vi "Utility_Read_Fluid_XML.vi"(11 "path":string) -> (3 "xmlout":string)   [LabVIEW 2016]
doc: "Reads pure fluid names from files in a given directory."
panel:
  out "Pure Fluids in REFPROP":string[][](table)=[["butene", "1-butene"], ["acetone", "propanone"], ["ammonia", "ammonia"], ["argon", "argon"], ["benzene", "benzene"], ["butane", "n-butane"], ["dodecane", "dodecane"], ["cis-butene", "cis-2-butene"], ["perfluorobutane", "decafluorobutane"], ["perfluoropentane", "dodecafluoropentane"], ["trifluoroiodomethane", "trifluoroiodomethane"], ["carbon monoxide", "carbon monoxide"], ["carbon dioxide", "carbon dioxide"], ["carbonyl sulfide", "carbon oxide sulfide"], ["cyclohexane", "cyclohexane"], ["cyclopropane", "cyclopropane"], ["deuterium", "deuterium"], ["heavy water", "deuterium oxide"], ["decane", "decane"], ["dimethylether", "ethylene oxide"], ["ethane", "ethane"], ["ethanol", "ethyl alcohol"], ["ethylene", "ethene"], ["fluorine", "fluorine"], ["hydrogen sulfide", "hydrogen sulfide"], ["helium", "helium-4"], ["heptane", "heptane"], ["hexane", "hexane"], ["hydrogen (normal)", "hydrogen (normal)"], ["isobutene", "2-methyl-1-propene"], ["isohexane", "2-methylpentane"], ["isopentane", "2-methylbutane"], ["isobutane", "2-methylpropane"], ["krypton", "krypton"], ["methane", "methane"], ["methanol", "methanol"], ["nitrous oxide", "dinitrogen monoxide"], ["neon", "neon"], ["neopentane", "2,2-dimethylpropane"], ["nitrogen trifluoride", "nitrogen trifluoride"], ["nitrogen", "nitrogen"], ["nonane", "nonane"], ["octane", "octane"], ["oxygen", "oxygen"], ["parahydrogen", "parahydrogen"], ["pentane", "pentane"], ["propane", "propane"], ["propylene", "propene"], ["propyne", "propyne"], ["R11", "trichlorofluoromethane"], ["R113", "1,1,2-trichloro-1,2,2-trifluoroethane"], ["R114", "1,2-dichloro-1,1,2,2-tetrafluoroethane"], ["R115", "chloropentafluoroethane"], ["R116", "hexafluoroethane"], ["R12", "dichlorodifluoromethane"], ["R123", "2,2-dichloro-1,1,1-trifluoroethane"], ["R124", "1-chloro-1,2,2,2-tetrafluoroethane"], ["R125", "pentafluoroethane"], ["R13", "chlorotrifluoromethane"], ["R134a", "1,1,1,2-tetrafluoroethane"], ["R14", "tetrafluoromethane"], ["R141b", "1,1-dichloro-1-fluoroethane"], ["R142b", "1-chloro-1,1-difluoroethane"], ["R143a", "1,1,1-trifluoroethane"], ["R152a", "1,1-difluoroethane"], ["R21", "dichlorofluoromethane"], ["R218", "octafluoropropane"], ["R22", "chlorodifluoromethane"], ["R227ea", "1,1,1,2,3,3,3-heptafluoropropane"], ["R23", "trifluoromethane"], ["R236ea", "1,1,1,2,3,3-hexafluoropropane"], ["R236fa", "1,1,1,3,3,3-hexafluoropropane"], ["R245ca", "1,1,2,2,3-pentafluoropropane"], ["R245fa", "1,1,1,3,3-pentafluoropropane"], ["R32", "difluoromethane"], ["R365mfc", "1,1,1,3,3-pentafluorobutane"], ["R41", "fluoromethane"], ["RC318", "octafluorocyclobutane"], ["sulfur hexafluoride", "sulfur hexafluoride"], ["sulfur dioxide", "sulfur dioxide"], ["trans-butene", "trans-2-butene"], ["toluene", "methylbenzene"], ["water", "water"], ["xenon", "xenon"]]
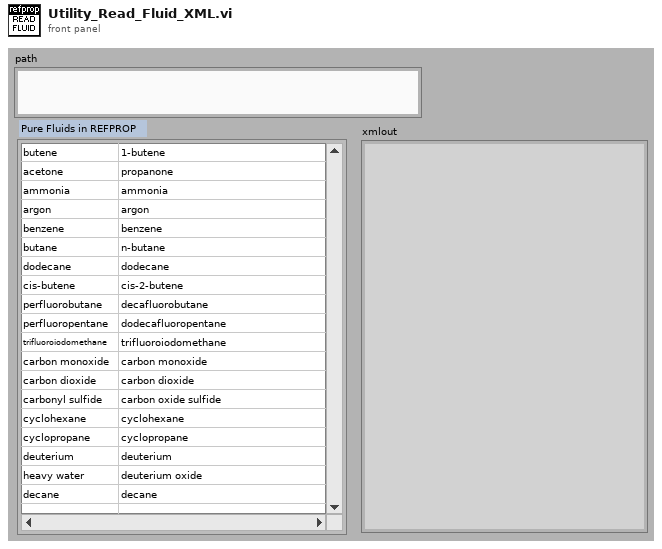
[diagram p1: front panel]
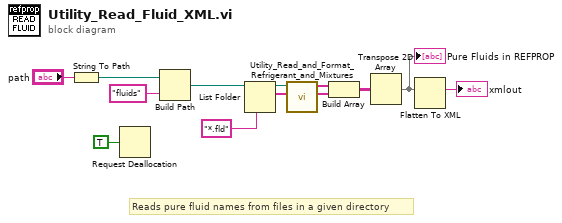
[diagram p0: block diagram]
diagram:
  # "Reads pure fluid names from files in a given directory"
  n1 = String To Path(string="path") -> (path=w6:path)
  n2 = Request Deallocation(TRUE ("标志")) -> ()
  n3 = Build Path(base path=w6, name or relative path="fluids") -> (appended path=w12:path)
  n4 = List Folder(path=w12, pattern="*.fld") -> (path out=w11:path, filenames=w10:string[])  [unwired: 2 in, 2 out]
  n5 = call "Utility_Read_and_Format_Refrigerant_and_Mixtures.vi"("File names"=w10, "Refprop Fluid or Mixture Directory"=w11) -> ("Refrigerant/Mixture Info"=w8:string[], "Refrigerant/Mixture Name"=w9:string[])  [unwired: 5 in, 1 out]
  n6 = Build Array(w9, w8) -> (w7:string[][])
  n7 = Transpose 2D Array(2D array=w7) -> (transposed array=w4:string[][])
  "Pure Fluids in REFPROP" <- w4
  n8 = Flatten To XML(anything=w4) -> (xml string=→"xmlout":string)
